vi "test10.vi"() -> ()   [LabVIEW 2018]
uses:
  test10.so
  <vilib>/Analysis/NI_AALBase.lvlib
  <vilib>/Utility/file.llb/Read Delimited Spreadsheet (DBL).vi
panel:
  out "raw_x_v":dbl[](array[numeric])
  out "conf_freq_f_v":dbl[](array[numeric])
  out "conf_v":dbl[](array[numeric])
  out "y_vv":dbl[][](array[numeric])
  out "Waveform Graph 3":dbl[](graph)
  out "Waveform Graph 2":dbl[](graph)
  out "Waveform Graph":dbl[](graph)
  out "error out 2":errorcluster
  out "arg4":dbl[](array[numeric])
  out "arg3":dbl[](array[numeric])
  out "return type":i32
  in  "arg1":dbl
  out "error out":errorcluster
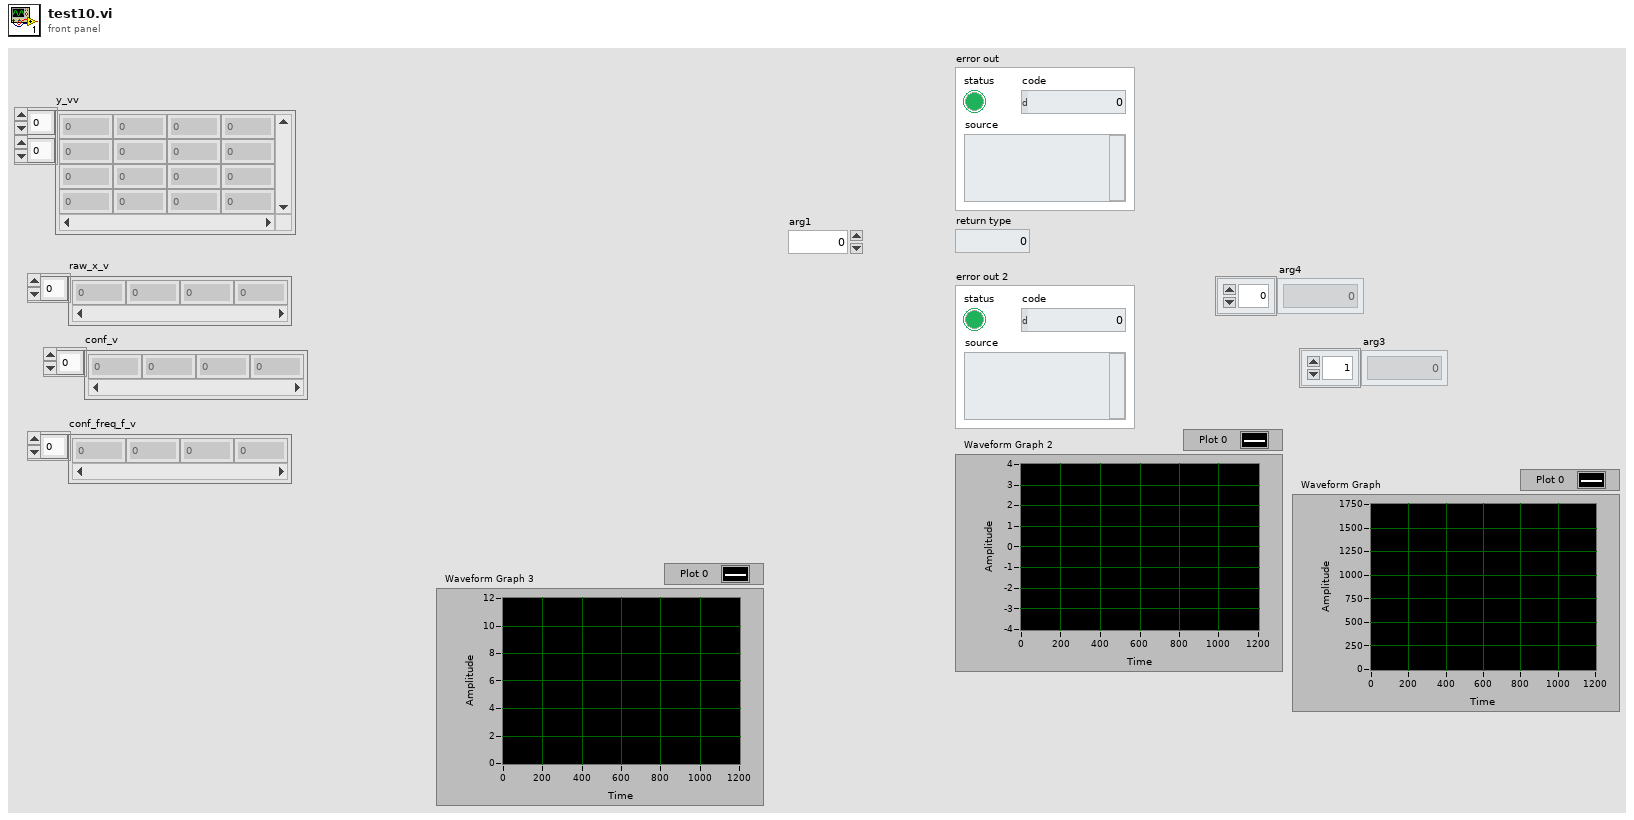
[diagram p1: front panel]
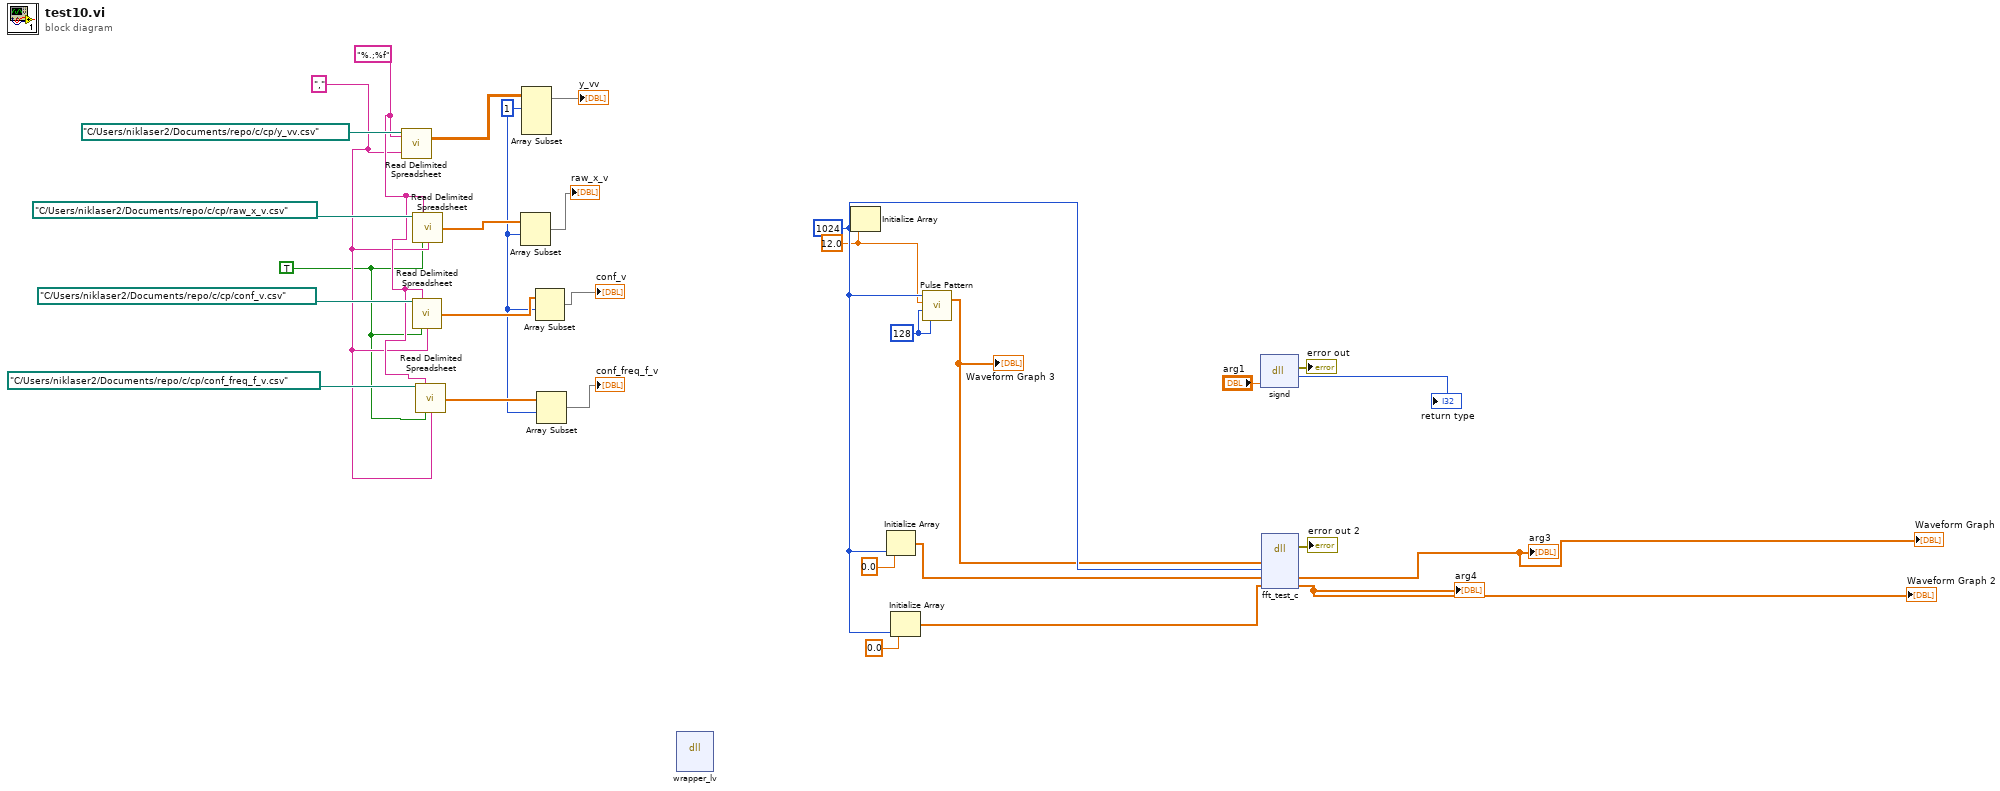
[diagram p0: block diagram]
diagram:
  w4 = 1 ("index")
  w1 = TRUE ("transpose? (F)")
  w12 = "%.;%f" ("format (%.3f)")
  w11 = "," ("delimiter (\\t)")
  w17 = 128 ("width")
  w19 = 12.0 ("element")
  w20 = 1024 ("dimension size")
  n1 = call-poly <vilib>:"Read Delimited Spreadsheet.vi"("file path (dialog if empty)"=path "C:/Users/niklaser2/Documents/repo/c/cp/y_vv.csv", "format (%.3f)"=w12, "delimiter (\\t)"=w11) -> ("all rows"=w10:dbl[][])  [unwired: 7 in, 5 out]
  n2 = call-poly <vilib>:"Read Delimited Spreadsheet.vi"("file path (dialog if empty)"=path "C:/Users/niklaser2/Documents/repo/c/cp/conf_v.csv", "format (%.3f)"=w12, "transpose? (F)"=w1, "delimiter (\\t)"=w11) -> ("first row"=w5:dbl[])  [unwired: 6 in, 5 out]
  n3 = call-poly <vilib>:"Read Delimited Spreadsheet.vi"("file path (dialog if empty)"=path "C:/Users/niklaser2/Documents/repo/c/cp/raw_x_v.csv", "format (%.3f)"=w12, "transpose? (F)"=w1, "delimiter (\\t)"=w11) -> ("first row"=w8:dbl[])  [unwired: 6 in, 5 out]
  n4 = call-poly <vilib>:"Read Delimited Spreadsheet.vi"("file path (dialog if empty)"=path "C:/Users/niklaser2/Documents/repo/c/cp/conf_freq_f_v.csv", "format (%.3f)"=w12, "transpose? (F)"=w1, "delimiter (\\t)"=w11) -> ("first row"=w6:dbl[])  [unwired: 6 in, 5 out]
  n5 = Array Subset(array=w8, index=w4) -> (→"raw_x_v":dbl[])  [unwired: 1 in]
  n6 = Array Subset(array=w10, index (row)=w4) -> (→"y_vv":dbl[][])  [unwired: 3 in]
  n7 = Array Subset(array=w5, index=w4) -> (→"conf_v":dbl[])  [unwired: 1 in]
  n8 = Array Subset(array=w6, index=w4) -> (→"conf_freq_f_v":dbl[])  [unwired: 1 in]
  n9 = dll-call lib="C:/Users/niklaser2/Documents/repo/c/cp/test10.so" fn="wrapper_lv"() -> ()  [unwired: 8 in, 2 out]
  n10 = Initialize Array(w19, w20) -> ()  [unwired: 1 out]
  n11 = Initialize Array(0.0 ("element"), w20) -> (w25:dbl[])
  n12 = Initialize Array(0.0 ("element"), w20) -> (w24:dbl[])
  n13 = call <vilib>:"Pulse Pattern.vi"("width"=w17, "delay"=w17, "amplitude"=w19, "samples"=w20) -> ("Pulse Pattern"=w18:dbl[])  [unwired: 1 out]
  "Waveform Graph 3" <- w18
  n14 = dll-call lib="C:/Users/niklaser2/Documents/repo/c/cp/test10.so" fn="signd"("arg1"="arg1") -> (error out=→"error out":errorcluster, "return type"=→"return type":i32)  [unwired: 4 in, 1 out]
  n15 = dll-call lib="C:/Users/niklaser2/Documents/repo/c/cp/test10.so" fn="fft_test_c"("arg1"=w18, "arg2"=w20, "arg3"=w25, "arg4"=w24) -> (error out=→"error out 2":errorcluster, "arg3"=→"arg3" →"Waveform Graph":dbl[], "arg4"=→"arg4" →"Waveform Graph 2":dbl[])  [unwired: 6 in, 1 out]
